vi "Get Wire Type.vi"(8 "error in (no error)":errorcluster, 11 "Scalar Encoder in":refnum<class "Scalar Type.lvclass">) -> (0 "error out":errorcluster, 2 "Wire Type":T1, 3 "Scalar Encoder out":refnum<class "Scalar Type.lvclass">)   [LabVIEW 2020, in "Protobuf RAW.lvlib" / "Scalar Type.lvclass"]
uses:
  Scalar Type.lvclass
  Type Serializer/Wire Type.ctl
  Wire Type Group/Wire Type Group.lvclass
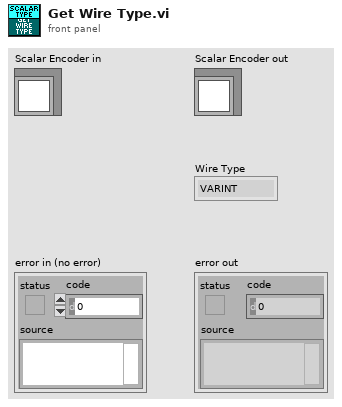
[diagram p1: front panel]
types:
  T1 = typedef "Protobuf RAW.lvlib/Wire Type Group.lvclass/Wire Type.ctl" = enum16{"VARINT", "I64", "LEN", "SGROUP", "EGROUP", "I32"}
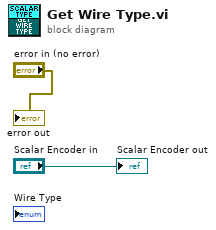
[diagram p0: block diagram]
diagram:
  "error out" <- "error in (no error)"
  "Scalar Encoder out" <- "Scalar Encoder in"
